vi "Global 1.vi"() -> ()   [LabVIEW 2023]
panel:
  out "counts":dbl
  in  "stop counter":bool
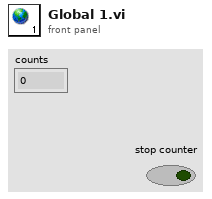
[diagram p1: front panel]
diagram:
